vi "FPGA Target, AI0 & AO0.vi"() -> ()   [LabVIEW 2018]
uses:
  <vilib>/rvi/eio/common/nirviEmuTemplateMethod_errors.vi
  <vilib>/rvi/interface/RandomDataEmulation/niFpgaRandomDataHandleErrors.vi
  <vilib>/eio/EIONode/EIONode.xnode
  <vilib>/rvi/DataTransferAndStorage/Container/XNode/niFpgaContainer.xnode
  <vilib>/rvi/interface/RandomDataEmulation/nirviRandomDataFpgaReadWriteTemplate.vi
panel:
  out "s? t:f":i16
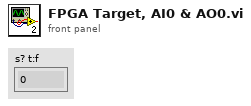
[diagram p1: front panel]
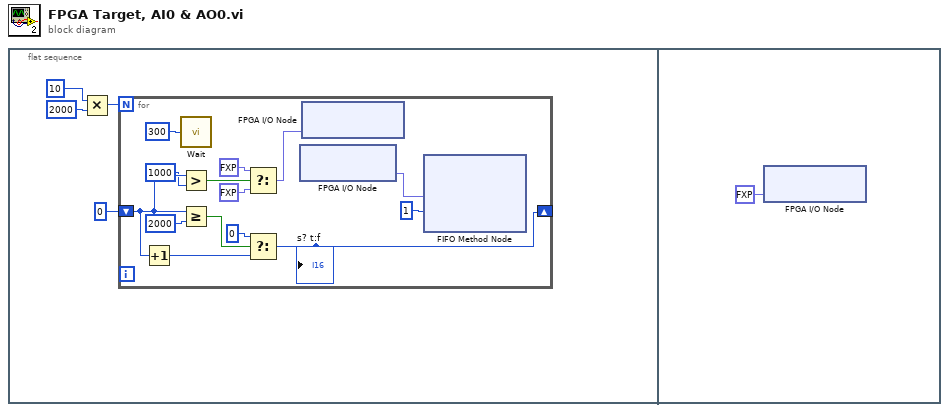
[diagram p0: block diagram]
diagram:
  n1 = flat-sequence {
    frame #0 {
      n2 = Multiply(x=10 ("Number of Loops"), y=2000) -> (x*y=w3:i32)
      n3 = for {
        N: w3 -> [_]
        shift-right: [w18] -> _
        shift-left: i16 0 -> [w8]
        n4 = Increment(x=w8) -> (x+1=w11:i16)
        n5 = call "Wait"("Count(uSec)"=u32 300) -> ()  [unwired: 1 out]
        n6 = Greater?(x=w8, y=i16 1000 ("x")) -> (0:w17:bool)
        n7 = Greater Or Equal?(x=w8, y=i16 2000) -> (x >= y?=w10:bool)
        n8 = Select(t=fxp<+/-,20,5> -5.0, s=w17, f=fxp<+/-,20,5> 0.0 ("Mod6/AO0")) -> (s? t:f=w6:fxp<+/-,20,5>)
        n9 = Select(t=i16 0, s=w10, f=w11) -> (s? t:f=w18:i16)
        "s? t:f" <- w18
        n10 = xnode "FPGA I/O Node"() -> ("Mod5/AI0"=w5:fxp<+/-,20,5>)  [unwired: 1 in, 1 out]
        n11 = xnode "FPGA I/O Node"("Mod6/AO0"=w6) -> ()  [unwired: 1 in, 1 out]
        n12 = xnode ("FIFO Method Node")("Element"=w5, "Timeout"=1) -> ()  [unwired: 1 in, 2 out]
      }
    }
    frame #1 {
      n13 = xnode "FPGA I/O Node"("Mod6/AO0"=fxp<+/-,20,5> 0.0) -> ()  [unwired: 1 in, 1 out]
    }
  }
